vi "Move Next Interval.vi"(8 "error in":errorcluster, 10 "Interval Token in":T1, 11 "Intervals in":T2[](array[typedef])) -> (0 "error out":errorcluster, 1 "Next interval time (ms)":u32, 2 "Interval Token out":T1, 3 "Intervals out":T2[](array[typedef]))   [LabVIEW 2021, in "Interval Timer.lvlib"]
doc: "Using 'Intervals in' and 'Interval Token in', calculate and track the current position in the software-timed interval sequence. Return a copy of 'Intervals in' to 'Intervals out', the future time coordinate when the next interval elapses to 'Next interval time (ms)', and the updated position to 'Interval Token out'. Designed for use in a loop."
uses:
  Interval Timer.lvlib
  Repeat Interval.ctl
  Interval Length.ctl
  Interval Token.ctl
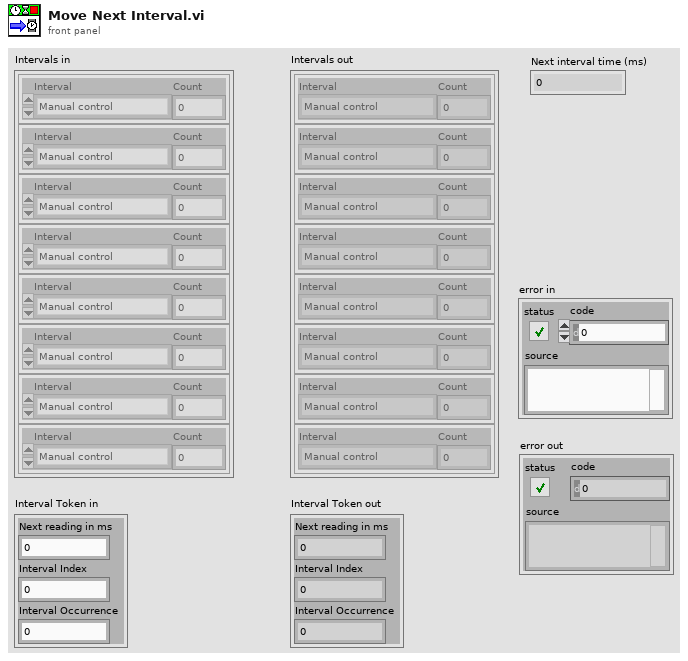
[diagram p1: front panel]
types:
  T1 = typedef "Interval Timer.lvlib/Interval Token.ctl" = cluster{"Next reading in ms":u32, "Interval Index":i32, "Interval Occurrence":i32}
  T2 = typedef "Interval Timer.lvlib/Repeat Interval.ctl" = cluster{"Interval":T3, "Count":i32}
  T3 = typedef "Interval Timer.lvlib/Interval Length.ctl" = enum16{"Manual control", "1 second", "10 seconds", "30 seconds", "60 seconds", "600 seconds", "1200 seconds", "3600 seconds"}
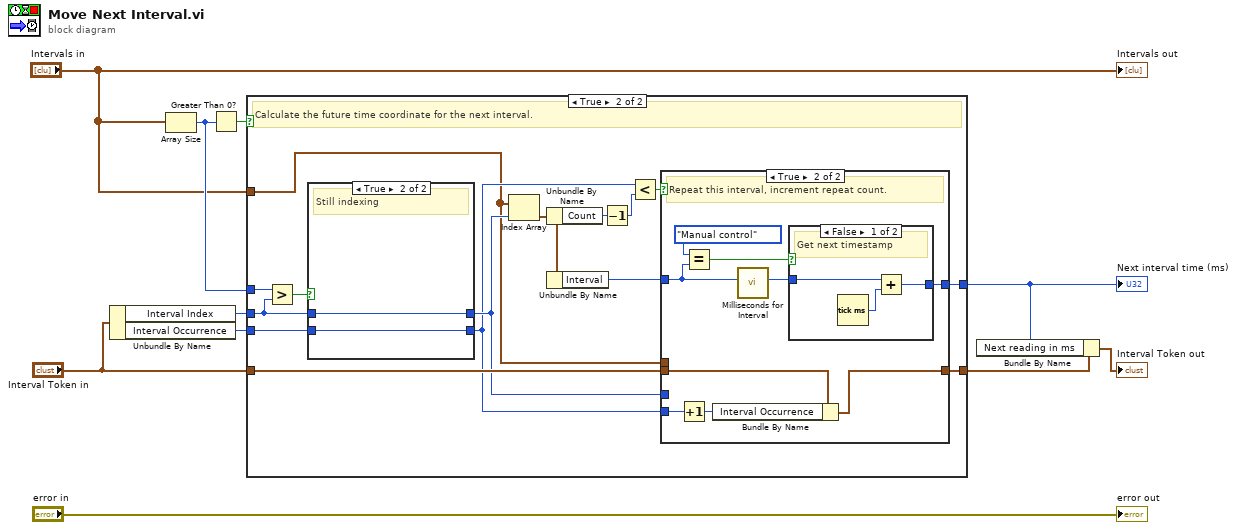
[diagram p0: block diagram]
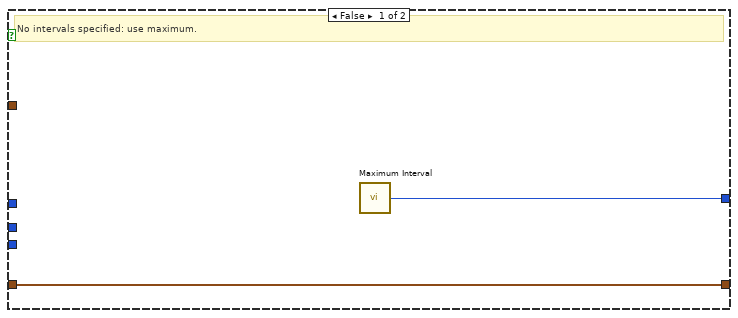
[diagram p2: hidden frame]
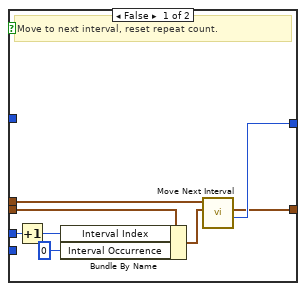
[diagram p3: hidden frame]
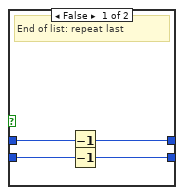
[diagram p5: hidden frame]
diagram:
  n1 = Unbundle By Name("Interval Token in") -> ("Interval Index"=w8:i32, "Interval Occurrence"=w9:i32)
  n2 = Array Size(array="Intervals in") -> (size(s)=w10:i32)
  n3 = Greater Than 0?(x=w10) -> (x > 0?=w5:bool)
  n4 = case shown="True" w5 {
    tunnel: w10 -> [_ w26]
    tunnel: w9 -> [_ w25]
    tunnel: w8 -> [_ w24]
    tunnel: "Interval Token in" -> [w12 w22]
    tunnel: [w11 w18] -> w2
    tunnel: [w12 w17] -> w3
    tunnel: "Intervals in" -> [_ w14]
    frame False {
      # "No intervals specified: use maximum."
      n5 = call "Maximum Interval.vi"() -> ("Maximum interval (ms)"=w11:u32)
    }
    frame True {
      # "Calculate the future time coordinate for the next interval."
      n6 = Greater?(x=w26, y=w24) -> (0:w27:bool)
      n7 = case shown="True" w27 {
        tunnel: w25 -> [w52 w53]
        tunnel: [w49 w54] -> w21
        tunnel: [w51 w53] -> w19
        tunnel: w24 -> [w50 w54]
        frame False {
          # "End of list: repeat last"
          n8 = Decrement(x=w50) -> (x-1=w49:i32)
          n9 = Decrement(x=w52) -> (x-1=w51:i32)
        }
        frame True {
          # "Still indexing"
        }
      }
      n10 = Index Array(array=w14, index=w21) -> (element=w15:T2)
      n11 = Unbundle By Name(w15) -> ("Count"=w16:i32)
      n12 = Unbundle By Name(w15) -> ("Interval"=w20:T3)
      n13 = Decrement(x=w16) -> (x-1=w13:i32)
      n14 = Less?(x=w19, y=w13) -> (x < y?=w23:bool)
      n15 = case shown="True" w23 {
        tunnel: w22 -> [w35 w44]
        tunnel: w21 -> [w33 _]
        tunnel: w20 -> [_ w39]
        tunnel: w19 -> [_ w42]
        tunnel: [w31 w41] -> w18
        tunnel: [w29 w37] -> w17
        tunnel: w14 -> [w28 _]
        frame False {
          # "Move to next interval, reset repeat count."
          n16 = Increment(x=w33) -> (x+1=w34:i32)
          n17 = Bundle By Name(cluster=w35, "Interval Index"=w34, "Interval Occurrence"=0) -> (w30:T1)
          n18 = call "Move Next Interval.vi"("Interval Token in"=w30, "Intervals in"=w28) -> ("Next interval time (ms)"=w31:u32, "Interval Token out"=w29:T1)  [unwired: 6 in, 2 out]
        }
        frame True {
          # "Repeat this interval, increment repeat count."
          n19 = Increment(x=w42) -> (x+1=w43:i32)
          n20 = Equal?(x=Interval_Length."Manual control" ("Interval"), y=w39) -> (x = y?=w40:bool)
          n21 = Bundle By Name(cluster=w44, "Interval Occurrence"=w43) -> (w37:T1)
          n22 = call "Milliseconds for Interval.vi"("Interval"=w39) -> ("Milliseconds"=w38:u32)  [unwired: 10 in]
          n23 = case shown="False" w40 {
            tunnel: [w46 w48] -> w41
            tunnel: w38 -> [w45 w48]
            frame False {
              # "Get next timestamp"
              n24 = Tick Count (ms)() -> (millisecond timer value=w47:u32)
              n25 = Add(x=w45, y=w47) -> (x+y=w46:u32)
            }
            frame True {
              # "Use special-case value"
            }
          }
        }
      }
    }
  }
  "Next interval time (ms)" <- w2
  n26 = Bundle By Name(cluster=w3, "Next reading in ms"=w2) -> (→"Interval Token out":T1)
  "Intervals out" <- "Intervals in"
  "error out" <- "error in"
